vi "sample true-false-indicator.vi"() -> ()   [LabVIEW 2013]
panel:
  out "s? t:f":i32
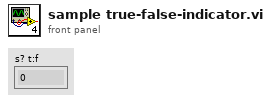
[diagram p1: front panel]
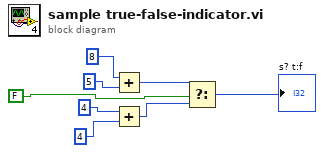
[diagram p0: block diagram]
diagram:
  n1 = Add(x=8, y=5) -> (x+y=w8:i32)
  n2 = Add(x=4, y=4) -> (x+y=w7:i32)
  n3 = Select(t=w8, s=FALSE, f=w7) -> (s? t:f=→"s? t:f":i32)
